vi "ScanAction.vi"(8 "error in (no error)":errorcluster caption="entrée d'erreur (pas d'erreur)", 9 "IndicePoint":i32, 11 "OR77200 en entrée":refnum<class "OR77200.lvclass"> caption="DNL_LabVIEW Object in") -> (0 "error out":errorcluster caption="sortie d'erreur", 2 "ScanParOut":dbl, 3 "OR77200 en sortie":refnum<class "OR77200.lvclass"> caption="DNL_LabVIEW Object out")   [LabVIEW 2010, in "OR77200.lvclass"]
uses:
  OR77200.lvclass
  OR77200.lvclass/OR77200.ctl
  BaseDevice/BaseDevice.lvclass
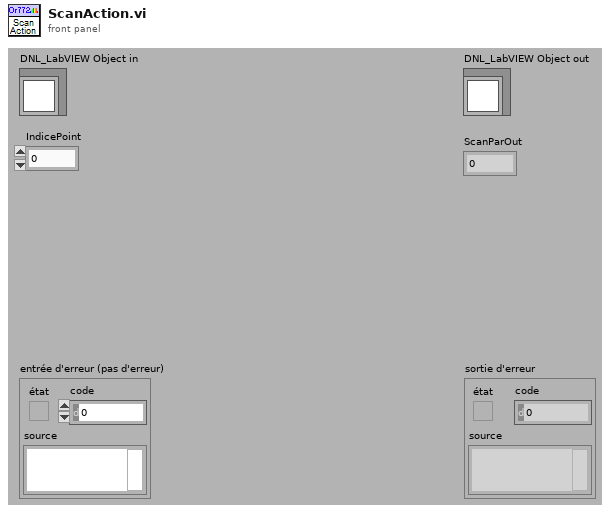
[diagram p1: front panel]
types:
  T1 = typedef "OR77200.lvclass/OR77200_Func.ctl" = enum16{"Position (nm)"}
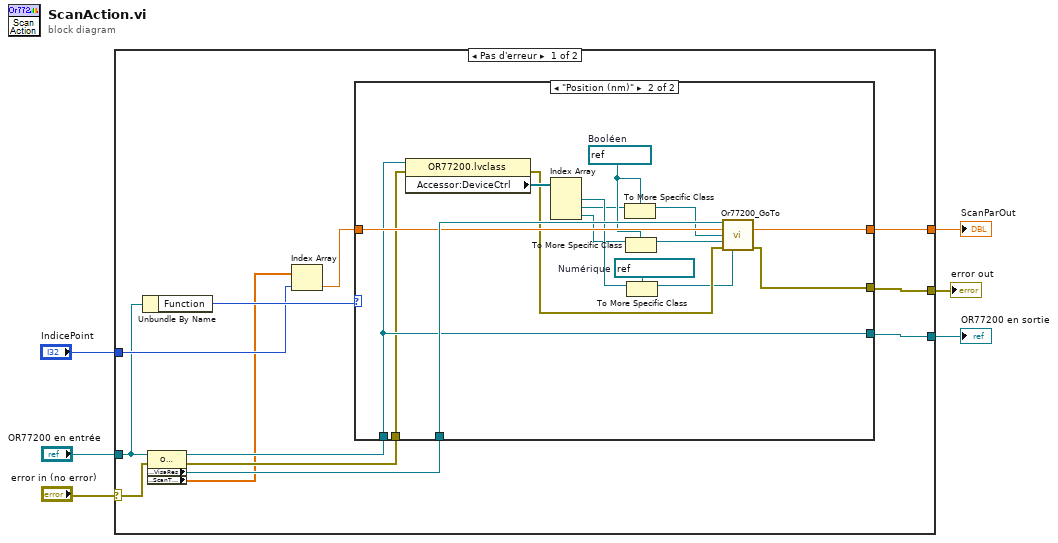
[diagram p0: block diagram]
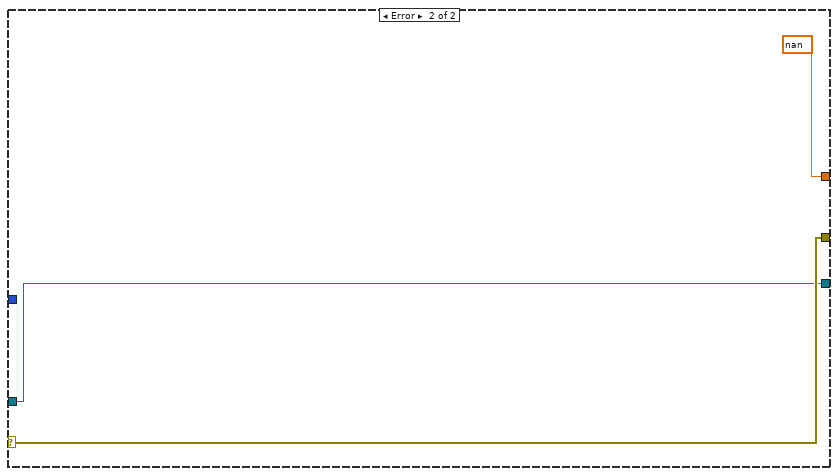
[diagram p3: hidden frame]
diagram:
  n1 = case shown="Pas d'erreur" "error in (no error)" {
    selector: "error in (no error)" -> [w18 w39]
    tunnel: "OR77200 en entrée" -> [w8 w38]
    tunnel: [w13 nan ("Lambda Out (nm)")] -> w4
    tunnel: [w14 w39] -> w3
    tunnel: [w16 w38] -> w2
    tunnel: "IndicePoint" -> [w10 _]
    frame No Error {
      n2 = Unbundle By Name(w8) -> ("Function"=w12:T1)
      n3 = property class="OR77200.lvclass"(reference=w8, error in=w18) -> (reference out=w17:refnum<class "OR77200.lvclass">, error out=w15:errorcluster, "Accessor:VisaRes"=w11:refnum<visa-resource-name>, "Accessor:ScanTable"=w7:dbl[])
      n4 = Index Array(array=w7, index=w10) -> (element=w9:dbl)
      n5 = case shown="\"Position (nm)\"" w12 {
        tunnel: w17 -> [w21 w33]
        tunnel: [w21 w33] -> w16
        tunnel: w15 -> [w20 w29]
        tunnel: [w20 w34] -> w14
        tunnel: w9 -> [w19 w36]
        tunnel: [w19 w35] -> w13
        tunnel: w11 -> [_ w37]
        frame Default {
        }
        frame "Position (nm)" {
          w25 = refnum<vi> refnum  # Numérique
          w30 = refnum<vi> refnum  # Booléen
          n6 = property class="OR77200.lvclass"(reference=w33, error in=w29) -> (error out=w28:errorcluster, "Accessor:DeviceCtrl"=w32:refnum<vi>[])  [unwired: 1 out]
          n7 = Index Array(array=w32) -> (element #1=w24:refnum<vi>, element #2=w22:refnum<vi>, element #3=w23:refnum<vi>)  [unwired: 3 in]
          n8 = To More Specific Class(target class=w30, reference=w22) -> (specific class reference=w31:refnum<vi>)  [unwired: 1 in, 1 out]
          n9 = To More Specific Class(target class=w30, reference=w23) -> (specific class reference=w27:refnum<vi>)  [unwired: 1 in, 1 out]
          n10 = To More Specific Class(target class=w25, reference=w24) -> (specific class reference=w26:refnum<vi>)  [unwired: 1 in, 1 out]
          n11 = call <userlib>:"Or77200_GoTo.vi"("Port"=w37, "Lambda (nm)"=w36, "Stop Ref"=w31, "Move Ref"=w27, "error In"=w28, "Lambda Ref"=w26) -> ("Lambda Out (nm)"=w35:dbl, "sortie d'erreur"=w34:errorcluster)  [unwired: 6 in, 2 out]
        }
      }
    }
    frame Error {
    }
  }
  "error out" <- w3
  "OR77200 en sortie" <- w2
  "ScanParOut" <- w4
